vi "Set DataType.vi"(8 "error in":errorcluster, 10 "Value":refnum<class "Value.lvclass">, 11 "Object Type in":refnum<class "Object Type Base.lvclass">) -> (0 "error out":errorcluster, 3 "Object Type out":refnum<class "Object Type Base.lvclass">)   [LabVIEW 2019, in "Electronic Datasheet.lvlib" / "Object Type Base.lvclass"]
uses:
  Object Type Base.lvclass
  Value/Value.lvclass
  Object Type Base.lvclass/Object Type Base.ctl
  Electronic Datasheet.lvlib
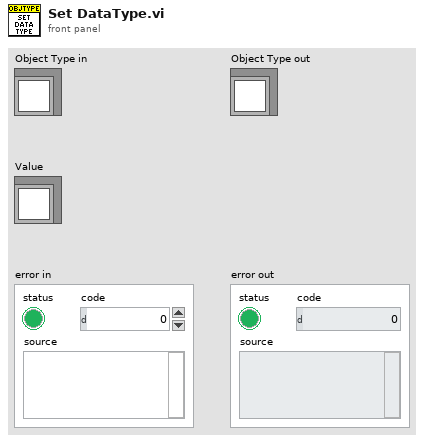
[diagram p1: front panel]
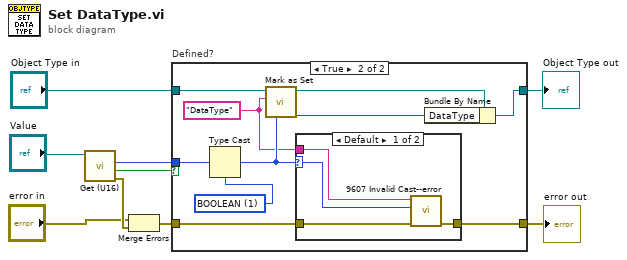
[diagram p0: block diagram]
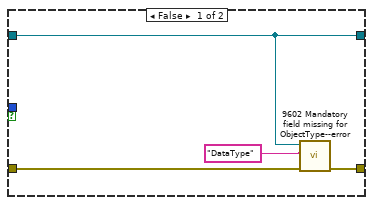
[diagram p2: hidden frame]
diagram:
  n1 = call "Get (U16).vi"("Value in"="Value") -> ("error out"=w3:errorcluster, "Defined?"=w6:bool, "Value"=w5:u16)  [unwired: 7 in, 1 out]
  n2 = Merge Errors("error in", w3) -> (w2:errorcluster)
  n3 = case "Defined?" shown="True" w6 {
    tunnel: "Object Type in" -> [w10 w22]
    tunnel: [w10 w21] -> w8
    tunnel: w5 -> [_ w19]
    tunnel: w2 -> [w13 w16]
    tunnel: [w12 w15] -> w4
    frame False {
      n4 = call "9602 Mandatory field missing for ObjectType--error.vi"("error in"=w13, "Field Name"="DataType" ("error message (\"\")"), "Object Type Base"=w10) -> ("error out"=w12:errorcluster)  [unwired: 8 in]
    }
    frame True {
      w18 = u16 1 items=["BOOLEAN"=1, "INTEGER8"=2, "INTEGER16"=3, "INTEGER32"=4, "UNSIGNED8"=5, "UNSIGNED16"=6, "UNSIGNED32"=7, "REAL32"=8, "VISIBLE_STRING"=9, "OCTET_STRING"=10, "UNICODE_STRING"=11, "TIME_OF_DAY"=12, "TIME_DIFFERENCE"=13, "RESERVED1"=14, "DOMAIN"=15, "INTEGER24"=16, "REAL64"=17, "INTEGER40"=18, "INTEGER48"=19, "INTEGER56"=20, "INTEGER64"=21, "UNSIGNED24"=22, "RESERVED2"=23, "UNSIGNED40"=24, "UNSIGNED48"=25, "UNSIGNED56"=26, "UNSIGNED64"=27, "RESERVED3"=28, "RESERVED4"=29, "RESERVED5"=30, "RESERVED6"=31, "PDO_COMMUNICATION_PARAMETER"=32, "PDO_MAPPING"=33, "SDO_PARAMETER"=34, "IDENTITY"=35, "RESERVED7"=36] ("DataType")
      w14 = "DataType" ("Field name")
      n5 = Type Cast(type=w18, x=w19) -> (*(type *) &x=w17:u16)
      n6 = call "Mark as Set.vi"("Field name"=w14, "Object Type in"=w22) -> ("Object Type out"=w20:refnum<class "Object Type Base.lvclass">)  [unwired: 9 in]
      n7 = case shown="Default" w17 {
        selector: w17 -> [w23 _]
        tunnel: w16 -> [w26 w27]
        tunnel: [w25 w27] -> w15
        tunnel: w14 -> [w24 _]
        frame Default {
          n8 = call "9607 Invalid Cast--error.vi"("error in"=w26, "Value"=w23, "Type"=w24) -> ("error out"=w25:errorcluster)  [unwired: 8 in]
        }
        frame 1..35 {
        }
      }
      n9 = Bundle By Name(cluster=w20, "DataType"=w17) -> (w21:refnum<class "Object Type Base.lvclass">)
    }
  }
  "Object Type out" <- w8
  "error out" <- w4
